vi "GL_SetAttribute.vi"(8 "No Error":errorcluster, 10 "Value":i32, 11 "GL Attribute":T1) -> (0 "Error Out":errorcluster)   [LabVIEW 2026, in "SDL3.lvlib" / "Video.lvlib"]
doc: "<B>Summary</B>\nSet an OpenGL window attribute before window creation.\n\n<B>Remarks</B>\nThis function sets the OpenGL attribute attr to value. The requested attributes should be set before creating an OpenGL window. You should use <B>SDL_GL_GetAttribute()</B> to check the values after creating the OpenGL context, since the values obtained can differ from the requested ones."
uses:
  Video.lvlib
  GLAttr--enum.ctl
  <vilib>/Utility/error.llb/Error Cluster From Error Code.vi
  Error/Error.lvlib
  Lib/SDL3.dll
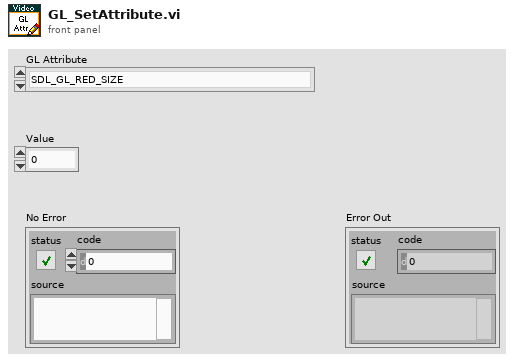
[diagram p1: front panel]
types:
  T1 = typedef "SDL3.lvlib/Video.lvlib/GLAttr--enum.ctl" = enum32{"SDL_GL_RED_SIZE", "SDL_GL_GREEN_SIZE", "SDL_GL_BLUE_SIZE", "SDL_GL_ALPHA_SIZE", "SDL_GL_BUFFER_SIZE", "SDL_GL_DOUBLEBUFFER", "SDL_GL_DEPTH_SIZE", "SDL_GL_STENCIL_SIZE", "SDL_GL_ACCUM_RED_SIZE", "SDL_GL_ACCUM_GREEN_SIZE", "SDL_GL_ACCUM_BLUE_SIZE", "SDL_GL_ACCUM_ALPHA_SIZE", "SDL_GL_STEREO", "SDL_GL_MULTISAMPLEBUFFERS", "SDL_GL_MULTISAMPLESAMPLES", "SDL_GL_ACCELERATED_VISUAL", "SDL_GL_RETAINED_BACKING", "SDL_GL_CONTEXT_MAJOR_VERSION", "SDL_GL_CONTEXT_MINOR_VERSION", "SDL_GL_CONTEXT_FLAGS", "SDL_GL_CONTEXT_PROFILE_MASK", "SDL_GL_SHARE_WITH_CURRENT_CONTEXT", "SDL_GL_FRAMEBUFFER_SRGB_CAPABLE", "SDL_GL_CONTEXT_RELEASE_BEHAVIOR", "SDL_GL_CONTEXT_RESET_NOTIFICATION", "SDL_GL_CONTEXT_NO_ERROR", "SDL_GL_FLOATBUFFERS", "SDL_GL_EGL_PLATFORM"}
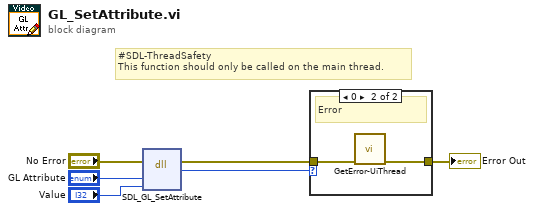
[diagram p0: block diagram]
diagram:
  # "#SDL-ThreadSafety\nThis function should only be called on the main thread."
  n1 = dll-call lib="C:/Users/saukko/Dev/LV-SDL3/Sources/SDL3/Lib/SDL3.*" fn="SDL_GL_SetAttribute"(error in="No Error", "attr"="GL Attribute", "value"="Value") -> (error out=w4:errorcluster, "return type"=w3:i32)  [unwired: 4 in, 1 out]
  n2 = case shown="0" w3 {
    tunnel: w4 -> [w7 w9]
    tunnel: [w7 w8] -> w5
    frame Default {
      # "Ok"
    }
    frame 0 {
      # "Error"
      n3 = call "GetError-UiThread.vi"("No Error"=w9) -> ("error out"=w8:errorcluster)  [unwired: 10 in]
    }
  }
  "Error Out" <- w5
